vi "Test Subscriber.vi"() -> ()   [LabVIEW 2021]
uses:
  ChannelCommon/typedef/FIFO Config.ctl
  ChannelCommon/ChannelCommon.lvlib
  CIFChannels/Typedef/Direction.ctl
  CIFChannels/CIFChannels.lvclass
  CIF_NIChn_Fifo_U8.lvclass
  ChannelCommon/typedef/New FIFO Instance Response.ctl
panel:
  out "U8 Data":u8[](array[numeric])
  in  "stop":bool
  out "timed out?":bool
  out "error out":errorcluster
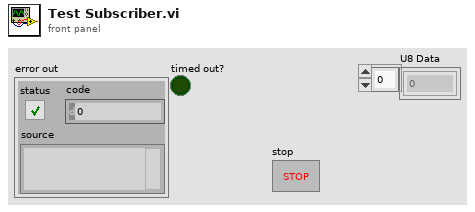
[diagram p1: front panel]
types:
  T1 = typedef "ChannelCommon.lvlib/New FIFO Instance Response.ctl" = cluster{"Publisher":string, "Custom Data":u8[]}
  T2 = typedef "ChannelCommon.lvlib/FIFO Config.ctl" = cluster{"Max Bytes/Msg":u64, "Max Msg/FIFO":u64, "Flags":u64}
  T3 = typedef "CIFChannels.lvclass/Direction.ctl" = enum16{"Publisher", "Subscriber"}
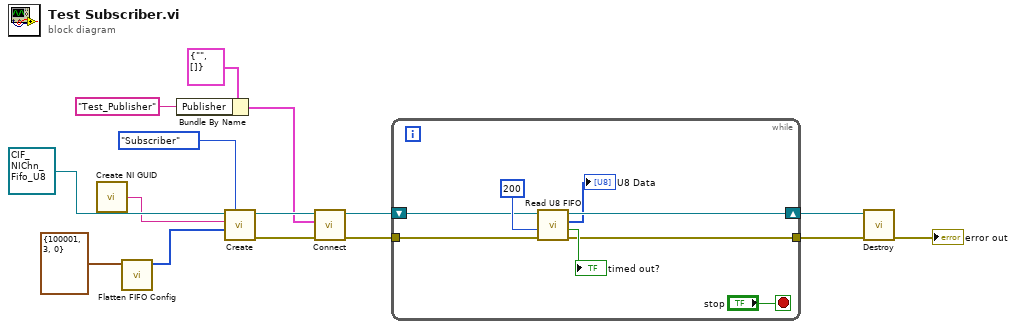
[diagram p0: block diagram]
diagram:
  n1 = call <vilib>:"Create NI GUID.vi"() -> ("NI GUID"=w9:string)
  n2 = call "Flatten FIFO Config.vi"("FIFO Config in"=T2 {"Max Bytes/Msg"=100001, "Max Msg/FIFO"=3, "Flags"=0}) -> ("Flattened FIFO Config"=w4:u8[])  [unwired: 10 in]
  n3 = Bundle By Name(cluster=T1 {"Publisher"="", "Custom Data"=[]} ("Connection"), "Publisher"="Test_Publisher" ("Connection Name")) -> (w1:T1)
  n4 = call-dynamic "Create.vi"("Direction"=Direction."Subscriber", "Custom Config Data"=w4, "Name"=w9, "CIFFIFO in"=refnum<class "CIF_NIChn_Fifo_U8.lvclass"> refnum ("CIF_NIChn_Fifo_Power.lvclass")) -> ("error out"=w12:errorcluster, "CIFFIFO out"=w13:refnum<class "CIF_NIChn_Fifo_U8.lvclass">)  [unwired: 6 in]
  n5 = call-dynamic "Connect.vi"("error in (no error)"=w12, "Connection"=w1, "CIFTag in"=w13) -> ("error out"=w6:errorcluster, "CIFTag out"=w8:refnum<class "CIF_NIChn_Fifo_U8.lvclass">)  [unwired: 7 in]
  n6 = while {
    shift-right: [w23] -> w15
    shift-left: w8 -> [w21]
    tunnel: w6 -> [w20]
    tunnel: [w18] -> w5
    stop <- "stop" stop-if-true
    n7 = call-dynamic "Read U8 FIFO.vi"("error in (no error)"=w20, "Timeout (ms)"=200, "CIFFIFO in"=w21) -> ("error out"=w18:errorcluster, "timed out?"=→"timed out?":bool, "Data out"=→"U8 Data":u8[], "CIFFIFO out"=w23:refnum<class "CIF_NIChn_Fifo_U8.lvclass">)  [unwired: 4 in, 1 out]
  }
  n8 = call-dynamic "Destroy.vi"("error in (no error)"=w5, "CIFFIFO in"=w15) -> ("error out"=→"error out":errorcluster)  [unwired: 8 in, 1 out]
